vi "str2boolen.vi"(1 "Str":string) -> (0 "Boolen":bool)   [LabVIEW 2014]
doc: "true、false"
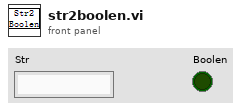
[diagram p1: front panel]
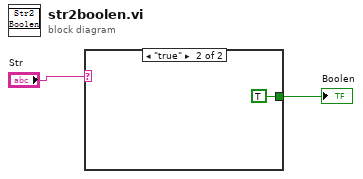
[diagram p0: block diagram]
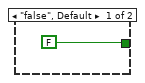
[diagram p2: hidden frame]
diagram:
  n1 = case shown="\"true\"" "Str" {
    tunnel: [FALSE TRUE] -> w1
    frame "false", Default {
    }
    frame "true" {
    }
  }
  "Boolen" <- w1
